vi "Inspect Tell.vi"(4 "Alias":string, 6 "Msg":refnum<class "Msg.lvclass">, 7 "Actor in":refnum<data-value>, 10 "Teller":T1 {"Absolute Time" format="%<%x %.3X>T"}) -> (0 "Error out":errorcluster, 5 "Actor out":refnum<data-value>)   [LabVIEW 2020, in "jettl.lvlib"]
uses:
  jettl.lvlib
  Actor/Actor.lvclass
  Msg/Msg.lvclass
  Msgs.ctl
  Layer.ctl
  Refs/Refs.lvclass
  Actor.ctl
  Relation.ctl
  Transport/Transport.lvclass
  Unified Layer.ctl
  Actor Attributes.ctl
  Teller.ctl
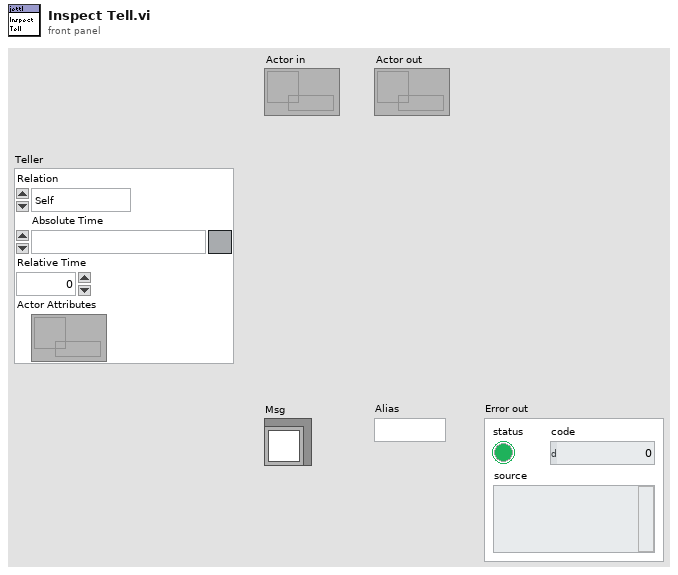
[diagram p1: front panel]
types:
  T1 = typedef "jettl.lvlib/Teller.ctl" = cluster{"Relation":T2, "Absolute Time":timestamp, "Relative Time":dbl, "Actor Attributes":refnum<data-value>}
  T2 = typedef "jettl.lvlib/Relation.ctl" = enum16{"Self", "Parent", "Child"}
  T3 = typedef "jettl.lvlib/Actor.ctl" = cluster{"Layer":T4, "Actor":refnum<class "Actor.lvclass">, "Refs":refnum<class "Refs.lvclass">}
  T4 = typedef "jettl.lvlib/Layer.ctl" = cluster{"Msgs":T5, "Leaf":bool, "Index":i32}
  T5 = typedef "jettl.lvlib/Msgs.ctl" = set{refnum<class "Msg.lvclass">}
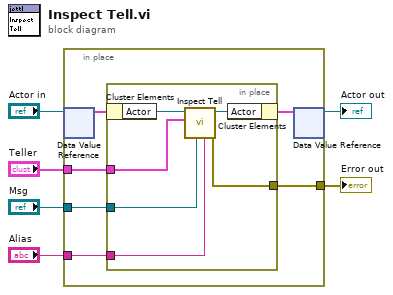
[diagram p0: block diagram]
diagram:
  n1 = in-place {
    in-place-border: [w10] -> w4
    in-place-border: "Msg" -> [w9]
    in-place-border: "Alias" -> [w8]
    in-place-border: "Teller" -> [w7]
    n2 = in-place-dvr #1("Actor in") -> (w12:T3)  [unwired: 1 out]
    n3 = in-place {
      in-place-border: [w16] -> w10
      in-place-border: w9 -> [w15]
      in-place-border: w8 -> [w14]
      in-place-border: w7 -> [w13]
      n4 = in-place-cluster #2(w12) -> ("Actor"=w18:refnum<class "Actor.lvclass">)
      n5 = call-dynamic "Inspect Tell.vi"("Alias"=w14, "Msg"=w15, "Teller"=w13, "Actor in"=w18) -> ("Error out"=w16:errorcluster, "Actor out"=w17:refnum<class "Actor.lvclass">)  [unwired: 6 in]
      n6 = in-place-cluster #2("Actor"=w17) -> (w11:T3)
    }
    n7 = in-place-dvr #1(w11) -> (→"Actor out":refnum<data-value>)  [unwired: 1 out]
  }
  "Error out" <- w4
